vi "QueryDeviceInfo.vi"(0 "DeviceIndex":i32 format="%.0x") -> (1 "Product ID":u32, 2 "Board Name":string, 3 "DIO Bytes":u32 format="%.0g", 4 "Counters":u32 format="%.0g")   [LabVIEW 2012]
doc: "This VI can be used to determine certain characteristic of ACCES USB boards."
uses:
  <vilib>/Utility/importsl/GetValueByPointer/datatype.ctl
  <vilib>/Utility/importsl/GetValueByPointer/GetValueByPointer.xnode
  Windows/System32/AIOUSB.dll
panel:
  out "Pointer":u32
  out "pNameSize":u32
  out "error out":errorcluster
  out "pName":string
  out "Return":u32
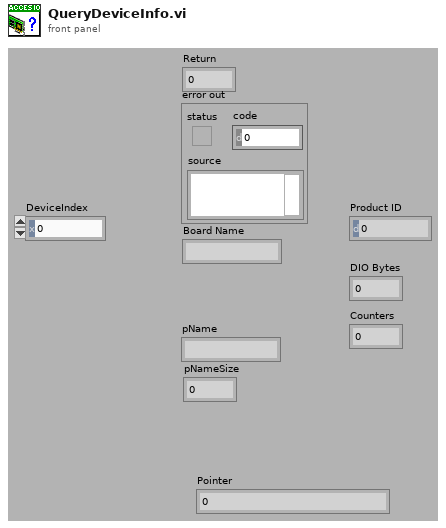
[diagram p1: front panel]
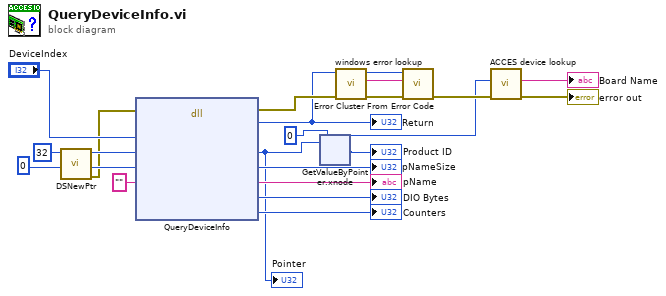
[diagram p0: block diagram]
diagram:
  n1 = call <vilib>:"DSNewPtr.vi"("Size"=u32 32) -> ("error out"=w10:errorcluster, "Pointer"=w11:u64)  [unwired: 9 in]
  n2 = dll-call lib="C:/Windows/System32/AIOUSB.dll" fn="QueryDeviceInfo"(error in=w10, "DeviceIndex"="DeviceIndex", "pPID"=w11, "pNameSize"=u32 0, "pName"="") -> (error out=w8:errorcluster, "return type"=w4:u32, "pPID"=w3:u32, "pNameSize"=→"pNameSize":u32, "pName"=→"pName":string, "pDIOBytes"=→"DIO Bytes":u32, "pCounters"=→"Counters":u32)  [unwired: 5 in, 1 out]
  "Return" <- w4
  "Pointer" <- w3
  n3 = xnode "GetValueByPointer.xnode"("Pointer"=w3, "InputType"=u32 0 ("Size")) -> ("Output"=w1:u32)  [unwired: 2 in, 1 out]
  "Product ID" <- w1
  n4 = call "windows error lookup.vi"("error in (no error)"=w8, "Error Code"=w4) -> ("error out"=w13:errorcluster, "error message (\"\")"=w5:string)  [unwired: 8 in]
  n5 = call <vilib>:"Error Cluster From Error Code.vi"("error in (no error)"=w13, "error message (\"\")"=w5, "error code (0)"=w4) -> ("error out"=w7:errorcluster)  [unwired: 6 in]
  n6 = call "ACCES device lookup.vi"("error in (no error)"=w7, "Device Code"=w1) -> ("error out"=→"error out":errorcluster, "error message (\"\")"=→"Board Name":string)  [unwired: 8 in]
